vi "LC Type Configuration.vi"() -> ()   [LabVIEW 2012]
uses:
  <vilib>/Utility/config.llb/Read Key (I32).vi
  <vilib>/Utility/config.llb/Write Key (U32).vi
  <vilib>/Utility/config.llb/NI_LVConfig.lvlib
panel:
  in  "Cancel":bool
  in  "LC Type":u16(ring) items=["No LC", "Spark"]
  in  "OK":bool
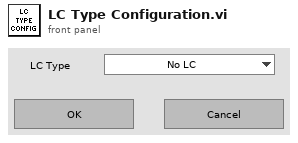
[diagram p1: front panel]
types:
  T1 = typedef "NI_LVConfig.lvlib/Config Data RefNum.ctl" = refnum<k1>
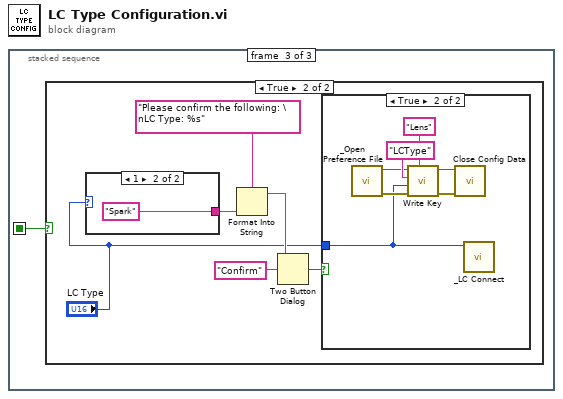
[diagram p0: block diagram]
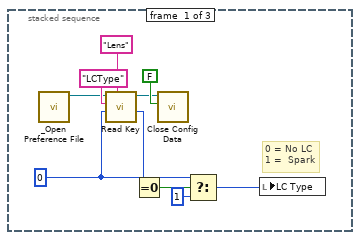
[diagram p2: hidden frame]
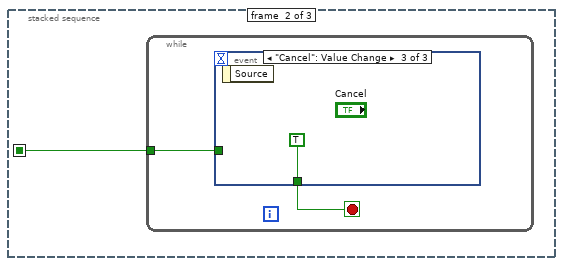
[diagram p3: hidden frame]
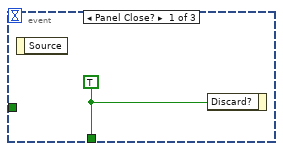
[diagram p4: hidden frame]
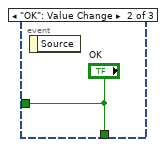
[diagram p5: hidden frame]
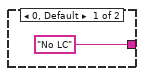
[diagram p7: hidden frame]
diagram:
  n1 = stacked-sequence {
    seq-local: [_ w11 _] -> [_ _ w17]
    frame #0 {
      w2 = 0 ("y")
      # "0 = No LC\n1 =  Spark"
      n2 = call "_Open Preference File.vi"() -> ("refnum"=w7:T1)  [unwired: 1 in, 6 out]
      n3 = call-poly <vilib>:"Read Key.vi"("section"="Lens", "default value"=w2, "key"="LCType" ("section"), "refnum"=w7) -> ("value"=w4:i32, "refnum out"=w6:T1)  [unwired: 1 in, 5 out]
      n4 = Equal To 0?(x=w4) -> (x = 0?=w3:bool)
      n5 = call <vilib>:"Close Config Data.vi"("write file if changed (T)"=FALSE ("write configuration file? (T)"), "refnum"=w6) -> ()  [unwired: 1 in, 9 out]
      n6 = Select(t=w2, s=w3, f=1) -> (s? t:f=w1:i32)
      n7 = local write "LC Type"(w1) -> ()
    }
    frame #1 {
      n8 = while {
        tunnel: [w12] -> w11
        stop <- w13 stop-if-true
        n9 = event shown="[2] \"Cancel\": Value Change" {
          selector: _ -> [_ _ _]
          dyn-events: _ -> [_ _ _]
          timeout: _ -> [_ _ _]
          tunnel: [w14 "OK" TRUE ("OK")] -> w13
          tunnel: [_ "OK" _] -> w12
          event Panel Close? {
            w14 = TRUE
            n10 = event-data() -> ()  [unwired: 2 out]
            n11 = event-data("Discard?"=w14) -> ()  [unwired: 1 in, 1 out]
          }
          event "OK": Value Change {
            n12 = event-data() -> ()  [unwired: 2 out]
          }
          event "Cancel": Value Change {
            n13 = event-data() -> ()  [unwired: 2 out]
          }
        }
      }
    }
    frame #2 {
      n14 = case shown="True" w17 {
        frame False {
        }
        frame True {
          n15 = case shown="1" "LC Type" {
            tunnel: ["No LC" "Spark"] -> w18
            frame 0, Default {
            }
            frame 1 {
            }
          }
          n16 = Format Into String(format string="Please confirm the following: \nLC Type: %s", w18) -> (resulting string=w21:string)  [unwired: 2 in, 1 out]
          n17 = Two Button Dialog(message=w21, 2:"Confirm" ("T button name (\"OK\")")) -> (T button?=w20:bool)  [unwired: 1 in]
          n18 = case shown="True" w20 {
            tunnel: "LC Type" -> [_ w26]
            frame False {
            }
            frame True {
              n19 = call "_Open Preference File.vi"() -> ("error"=w27:errorcluster, "refnum"=w28:T1)  [unwired: 1 in, 5 out]
              n20 = call-poly <vilib>:"Write Key.vi"("section"="Lens", "error in (no error)"=w27, "value"=w26, "key"="LCType" ("section"), "refnum"=w28) -> ("error out"=w29:errorcluster, "refnum out"=w30:T1)  [unwired: 5 out]
              n21 = call <vilib>:"Close Config Data.vi"("error in (no error)"=w29, "refnum"=w30) -> ()  [unwired: 1 in, 9 out]
              n22 = call "_LC Connect.vi"("LC Type"=w26) -> ()  [unwired: 7 out]
            }
          }
        }
      }
    }
  }
